vi "剖面数据模拟器.vi"() -> ()   [LabVIEW 2016]
uses:
  <vilib>/Utility/miscctls.llb/LVPointTypeDef.ctl
panel:
  out "缓存":T1[](array[typedef])
  out "data":T1
  in  "Tabe Name":string
  in  "错误输入（无错误）":errorcluster
  out "错误输出":errorcluster
  in  "数据库类型":T2
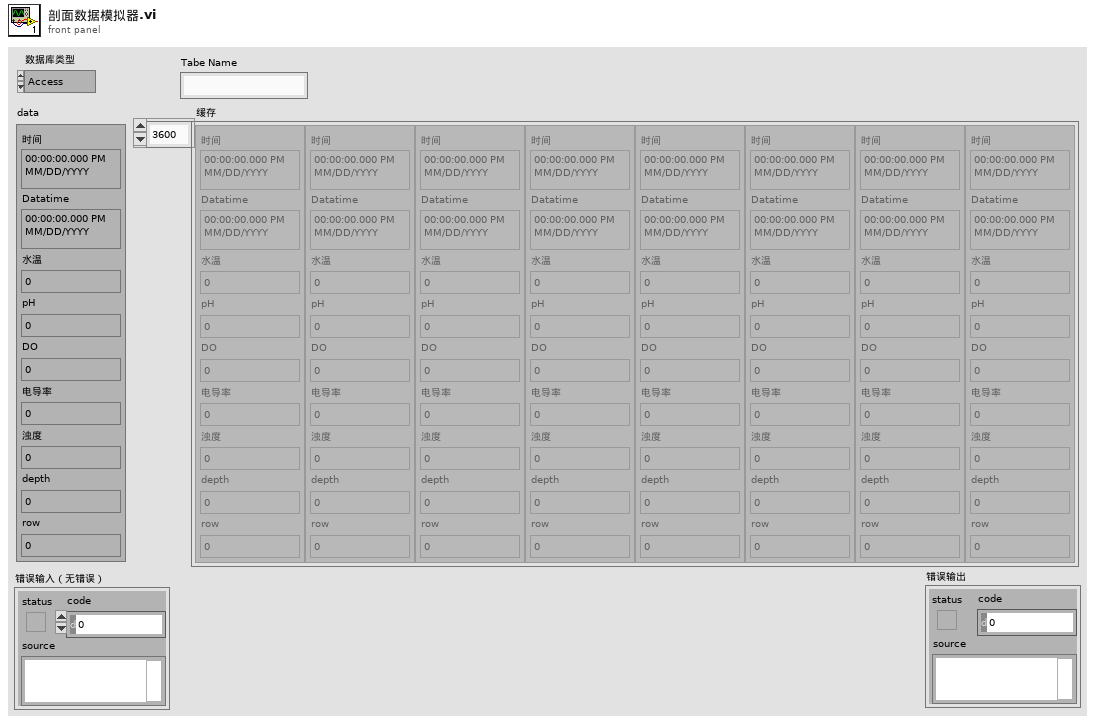
[diagram p1: front panel]
types:
  T1 = typedef "剖面数据字段定义.ctl" = cluster{"时间":timestamp, "Datatime":timestamp, "水温":sgl, "pH":sgl, "DO":sgl, "电导率":sgl, "浊度":sgl, "depth":sgl, "row":u32}
  T2 = typedef "数据库类型.ctl" = enum16{"Access", "SQLite"}
  T3 = typedef "LVPointTypeDef.ctl" = cluster{"Horizontal":i16, "Vertical":i16}
  T4 = typedef "LVDateTimeRec.ctl" = cluster{"秒数的小数部分":dbl, "秒":i32, "分":i32, "时":i32, "日":i32, "月":i32, "年":i32, "天数（周）":i32, "天数（年）":i32, "DST":i32}
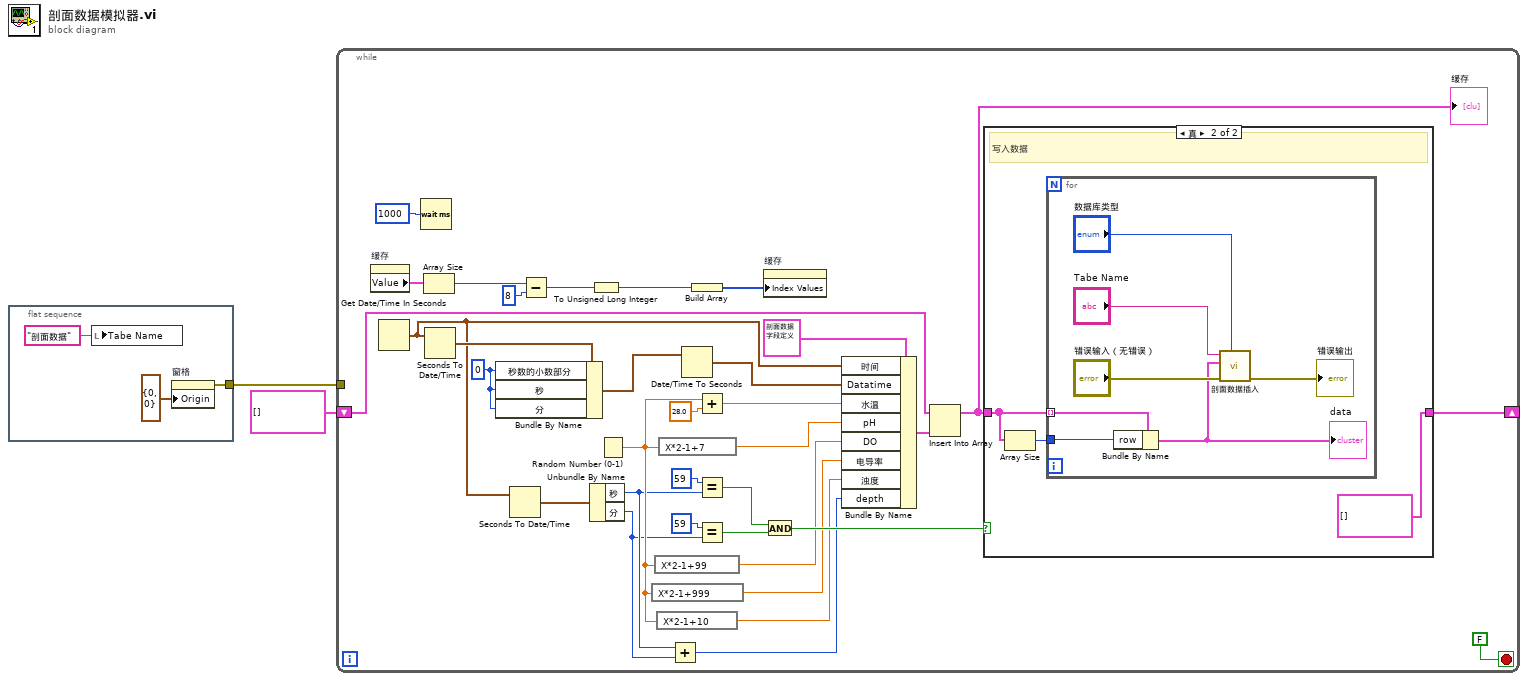
[diagram p0: block diagram]
diagram:
  n1 = flat-sequence {
    tunnel: [w4] -> w2
    frame #0 {
      n2 = local write "Tabe Name"("剖面数据" ("Tabe Name")) -> ()
      n3 = property on="窗格" class="Pane"("Origin"=T3 {"Horizontal"=0, "Vertical"=0} ("原点")) -> (error out=w4:errorcluster)  [unwired: 2 in, 1 out]
    }
  }
  n4 = while {
    tunnel: w2 -> [_]
    shift-right: [w17] -> _
    shift-left: T1[] [] -> [w33]
    stop <- FALSE stop-if-true
    w28 = 0 ("秒")
    n5 = property on="缓存" class="Arr (严格)"() -> ("Value"=w13:T1[])  [unwired: 2 in, 2 out]
    n6 = Get Date/Time In Seconds() -> (seconds since 1Jan1904=w25:timestamp)
    n7 = Wait (ms)(milliseconds to wait=u32 1000 ("等待时间（毫秒）")) -> ()  [unwired: 1 out]
    n8 = Array Size(array=w13) -> (size(s)=w12:i32)
    n9 = Seconds To Date/Time(time stamp (now)=w25) -> (date time rec=w29:T4)  [unwired: 1 in]
    n10 = Bundle By Name(cluster=w29, "秒数的小数部分"=w28, "秒"=w28, "分"=w28) -> (w26:T4)
    n11 = Seconds To Date/Time(time stamp (now)=w25) -> (date time rec=w30:T4)  [unwired: 1 in]
    n12 = Subtract(x=w12, y=8) -> (x-y=w10:i32)
    n13 = Unbundle By Name(w30) -> ("秒"=w16:i32, "分"=w15:i32)
    n14 = To Unsigned Long Integer(number=w10) -> (unsigned 32bit integer=w9:u32)
    n15 = Random Number (0-1)() -> (number: 0 to 1=w19:dbl)
    n16 = expression code="X*2-1+999"(w19) -> (w20:dbl)
    n17 = expression code="X*2-1+99"(w19) -> (w21:dbl)
    n18 = expression code="X*2-1+10"(w19) -> (w18:dbl)
    n19 = expression code="X*2-1+7"(w19) -> (w22:dbl)
    n20 = Add(x=w16, y=w15) -> (x+y=w14:i32)
    n21 = Date/Time To Seconds(2:w26) -> (0:w27:timestamp)  [unwired: 1 in]
    n22 = Build Array(w9) -> (w8:u32[])
    n23 = Add(x=w19, y=28.0) -> (x+y=w23:dbl)
    n24 = Equal?(x=59, y=w16) -> (x = y?=w37:bool)
    n25 = Equal?(x=59, y=w15) -> (x = y?=w36:bool)
    n26 = property on="缓存" class="Arr (严格)"("Index Values"=w8) -> ()  [unwired: 2 in, 2 out]
    n27 = And(x=w37, y=w36) -> (x .and. y?=w35:bool)
    n28 = Bundle By Name(cluster=T1 {"时间"=timestamp(0 s since 1904-01-01), "Datatime"=timestamp(0 s since 1904-01-01), "水温"=0.0, "pH"=0.0, "DO"=0.0, "电导率"=0.0, "浊度"=0.0, "depth"=0.0, "row"=0} ("data"), "时间"=w25, "Datatime"=w27, "水温"=w23, "pH"=w22, "DO"=w21, "电导率"=w20, "浊度"=w18, "depth"=w14) -> (w31:T1)
    n29 = Insert Into Array(array=w33, new element=w31) -> (w34:T1[])  [unwired: 1 in]
    "缓存" <- w34
    n30 = case shown="真" w35 {
      tunnel: w34 -> [w40 w42]
      tunnel: [w40 T1[] []] -> w17
      frame False {
      }
      frame True {
        # "写入数据"
        n31 = Array Size(array=w42) -> (size(s)=w41:i32)
        n32 = for {
          tunnel: w42 -> [w46] mode=indexing
          tunnel: w41 -> [w45]
          n33 = Bundle By Name(cluster=w46, "row"=w45) -> (w44:T1)
          "data" <- w44
          n34 = call "剖面数据插入.vi"("Tabe Name"="Tabe Name", "data"=w44, "错误输入（无错误）"="错误输入（无错误）", "数据库类型"="数据库类型") -> ("错误输出"=→"错误输出":errorcluster)  [unwired: 6 in]
        }
      }
    }
  }
